vi "Channel(s) Array to Channel(s) String.vi"(8 "error in (no error)":errorcluster, 10 "Channel(s)":i32[](array[numeric]), 11 "PXIe5413 in":refnum<class "PXIe5413.lvclass">) -> (0 "error out":errorcluster, 2 "Channels String":string, 3 "PXIe5413 out":refnum<class "PXIe5413.lvclass">)   [LabVIEW 2018, in "PXIe5413.lvlib" / "PXIe5413.lvclass"]
uses:
  PXIe5413.lvclass
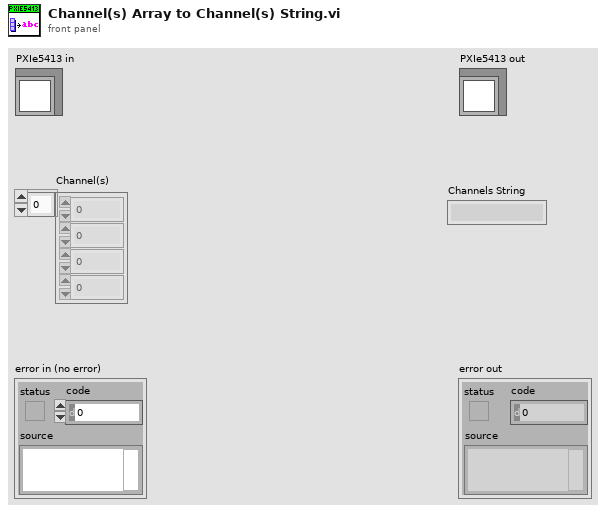
[diagram p1: front panel]
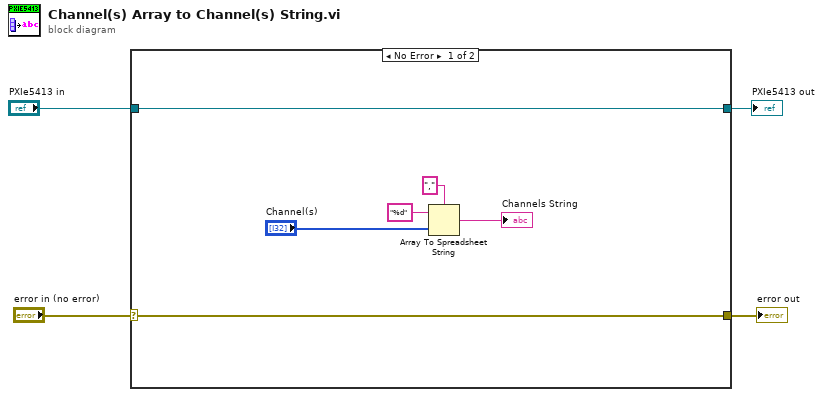
[diagram p0: block diagram]
diagram:
  n1 = case shown="No Error" "error in (no error)" {
    selector: "error in (no error)" -> [w9 w12]
    tunnel: [w9 w12] -> w3
    tunnel: [w10 w11] -> w1
    tunnel: "PXIe5413 in" -> [w10 w11]
    frame No Error {
      n2 = Array To Spreadsheet String(delimiter (Tab)=",", array="Channel(s)", 3:"%d" ("delimiter (Tab)")) -> (spreadsheet string=→"Channels String":string)
    }
    frame Error {
    }
  }
  "error out" <- w3
  "PXIe5413 out" <- w1
